vi "Set Light (reference).vi"(7 "Light State":enum16{"Inherit Value", "Off", "On"}(ring), 8 "error in (no error)":errorcluster, 9 "Position":T1, 10 "Light Refnum In":refnum<vi>, 11 "Scene Object In":refnum<vi>) -> (0 "error out":errorcluster, 2 "Light Refnum Out":refnum<vi>, 3 "Scene Object Out":refnum<vi>)   [LabVIEW 2020, in "NI_3D Picture Control.lvlib"]
doc: "Creates and positions a light source in 3D space relative to a 3D object."
uses:
  <vilib>/picture/3D Picture Control/NI_3D Picture Control.lvlib
  <vilib>/Utility/miscctls.llb/LV3DPointTypeDef.ctl
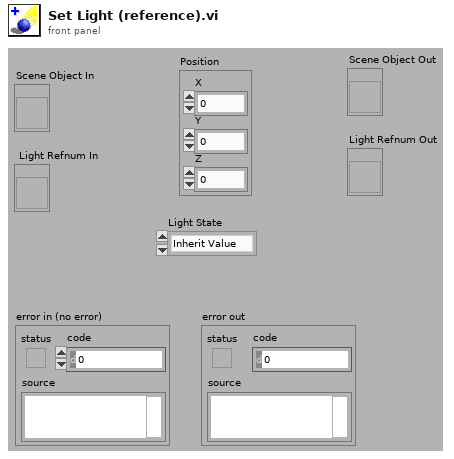
[diagram p1: front panel]
types:
  T1 = typedef "LV3DPointTypeDef.ctl" = cluster{"X":sgl, "Y":sgl, "Z":sgl}
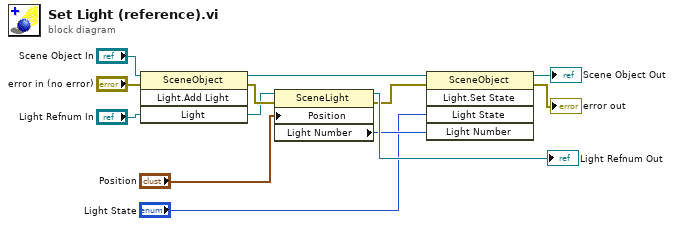
[diagram p0: block diagram]
diagram:
  n1 = invoke class="SceneObject" method="Light.Add Light"(reference="Scene Object In", error in="error in (no error)", "Light"="Light Refnum In") -> (reference out=w7:refnum<vi>, error out=w10:errorcluster, "Light"=w9:refnum<vi>)  [unwired: 1 in, 1 out]
  n2 = property class="SceneLight"(reference=w9, error in=w10, "Position"="Position") -> (reference out=→"Light Refnum Out":refnum<vi>, error out=w2:errorcluster, "Light Number"=w5:i32)
  n3 = invoke class="SceneObject" method="Light.Set State"(reference=w7, error in=w2, "Light State"="Light State", "Light Number"=w5) -> (reference out=→"Scene Object Out":refnum<vi>, error out=→"error out":errorcluster)  [unwired: 1 in, 3 out]
